vi "Left LIDAR (SubVI).vi"(11 "Refnum in":refnum<k20>) -> (0 "ft":dbl, 1 "in":dbl, 2 "cm":dbl, 3 "Refnum out":refnum<k20>)   [LabVIEW 2015]
uses:
  <vilib>/Utility/error.llb/Error Cluster From Error Code.vi
  <vilib>/rvi/errors/niLvFpgaAdjustHostInterfaceError.vi
  <vilib>/rvi/interface/nirviReadWriteControl/nirviReadWriteControl.xnode
  NiFpgaLv.dll
  <vilib>/rvi/interface/Simulation/niFpgaSimulationCallBeginRW.vi
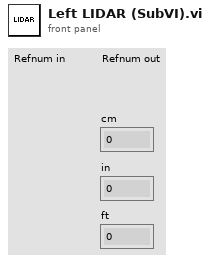
[diagram p1: front panel]
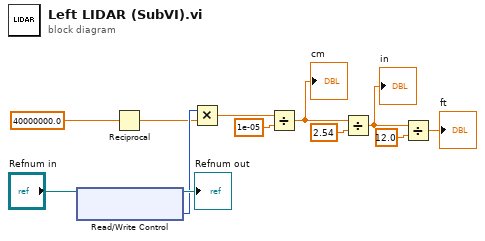
[diagram p0: block diagram]
diagram:
  n1 = xnode "Read/Write Control"("FPGA VI Reference In"="Refnum in") -> ("FPGA VI Reference Out"=→"Refnum out":refnum<k20>, "Pulse width ticks"=w3:u32)  [unwired: 1 in, 1 out]
  n2 = Reciprocal(x=40000000.0) -> (1/x=w2:dbl)
  n3 = Multiply(x=w3, y=w2) -> (x*y=w4:dbl)
  n4 = Divide(x=w4, y=1e-05) -> (x/y=w6:dbl)
  "cm" <- w6
  n5 = Divide(x=w6, y=2.54) -> (x/y=w10:dbl)
  "in" <- w10
  n6 = Divide(x=w10, y=12.0) -> (x/y=→"ft":dbl)
